vi "RP Lockin Batch Sweeper.vi"(6 "Samples per read":i32=1024, 8 "Error In":errorcluster, 9 "Dwell time":dbl=0.01, 10 "Frequencies":dbl[](array[numeric]), 11 "connection ID":refnum<k5>) -> (0 "Error Out":errorcluster, 1 "Y":dbl[](array[numeric]), 2 "X":dbl[](array[numeric]), 3 "connection ID out":refnum<k5>, 4 "F":dbl[](array[numeric]))   [LabVIEW 2015]
panel:
  out "32bit integer":i32
  out "Fifo cnt":i32
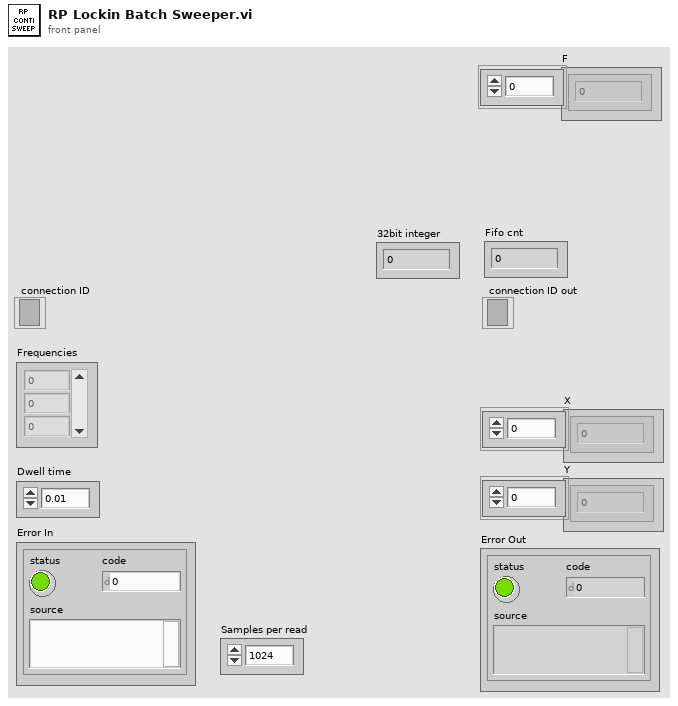
[diagram p1: front panel]
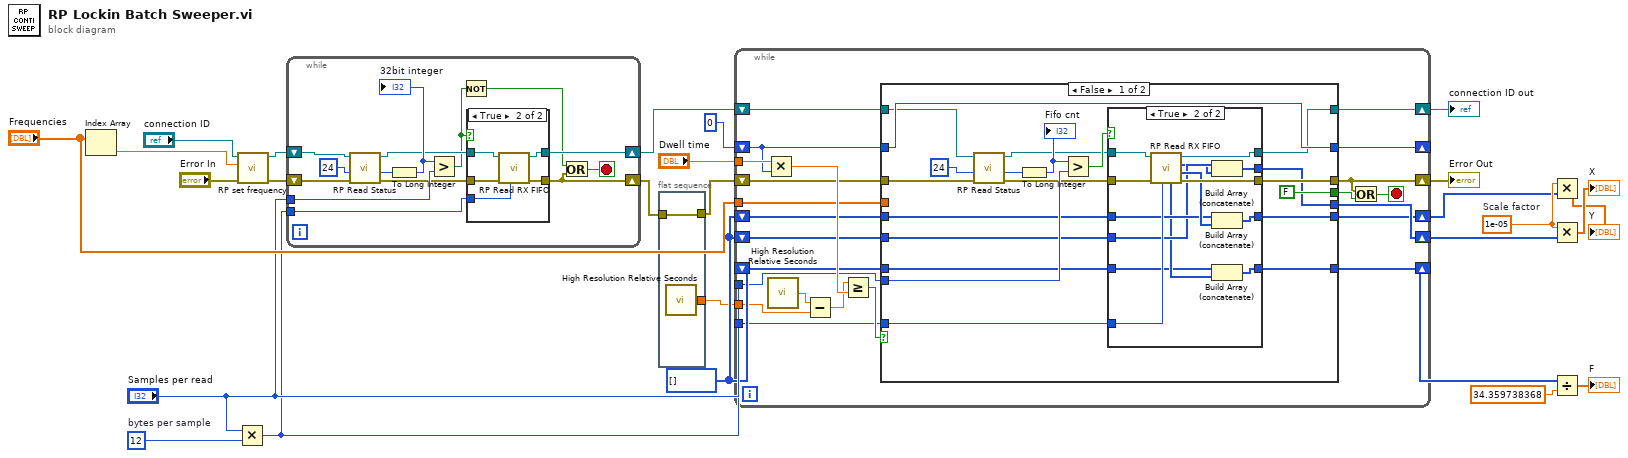
[diagram p0: block diagram]
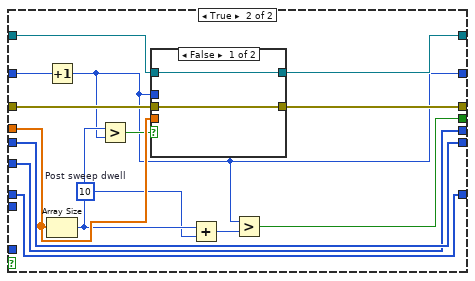
[diagram p4: hidden frame]
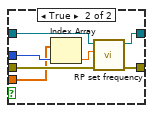
[diagram p5: hidden frame]
diagram:
  w12 = 1e-05  # Scale factor
  w9 = i32[] [] ("x*y")
  w20 = 12  # bytes per sample
  n1 = Index Array(array="Frequencies") -> (element=w24:dbl)  [unwired: 1 in]
  n2 = Multiply(x="Samples per read", y=w20) -> (x*y=w13:i32)
  n3 = call "RP set frequency.vi"("Error In"="Error In", "Frequency"=w24, "connection ID"="connection ID") -> ("Error Out"=w14:errorcluster, "connection ID out"=w16:refnum<k5>)  [unwired: 6 in, 1 out]
  n4 = while {
    tunnel: "Samples per read" -> [w37]
    shift-right: [w27] -> w3
    shift-left: w14 -> [w34]
    shift-right: [w32] -> w15
    shift-left: w16 -> [w33]
    tunnel: w13 -> [w31]
    stop <- w30 stop-if-true
    n5 = call "RP Read Status.vi"("Error In"=w34, "Status offset"=u64 24, "connection ID"=w33) -> ("Error Out"=w29:errorcluster, "Status response"=w38:u32, "connection ID out"=w36:refnum<k5>)  [unwired: 6 in]
    n6 = To Long Integer(number=w38) -> (32bit integer=w39:i32)
    "32bit integer" <- w39
    n7 = Greater?(x=w39, y=w37) -> (0:w35:bool)
    n8 = Not(x=w35) -> (.not. x?=w28:bool)
    n9 = case shown="True" w35 {
      tunnel: w36 -> [w42 w47]
      tunnel: w29 -> [w41 w46]
      tunnel: [w41 w45] -> w27
      tunnel: [w42 w44] -> w32
      tunnel: w31 -> [_ w43]
      frame False {
      }
      frame True {
        n10 = call "RP Read RX FIFO.vi"("FIFO Bytes per read"=w43, "Error In"=w46, "connection ID"=w47) -> ("Error Out"=w45:errorcluster, "connection ID out"=w44:refnum<k5>)  [unwired: 4 in, 3 out]
      }
    }
    n11 = Or(x=w28, y=w27) -> (x .or. y?=w30:bool)
  }
  n12 = flat-sequence {
    tunnel: w3 -> [w49]
    tunnel: [w49] -> w2
    tunnel: [w48] -> w1
    frame #0 {
      n13 = call <vilib>:"High Resolution Relative Seconds.vi"() -> ("relative seconds"=w48:dbl)
    }
  }
  n14 = while {
    shift-right: [w64] -> _
    shift-left: 0 -> [w66]
    tunnel: "Dwell time" -> [w72]
    tunnel: w1 -> [w68]
    tunnel: "Frequencies" -> [w65]
    shift-right: [w61] -> w10
    shift-left: w9 -> [w53]
    shift-right: [w52] -> w11
    shift-left: w9 -> [w60]
    tunnel: "Samples per read" -> [w63]
    tunnel: w13 -> [w62]
    shift-right: [w54] -> w18
    shift-left: w2 -> [w59]
    shift-right: [w57] -> w19
    shift-left: w15 -> [w58]
    shift-right: [w50] -> w7
    shift-left: w9 -> [w51]
    stop <- w55 stop-if-true
    n15 = Multiply(x=w72, y=w66) -> (x*y=w71:dbl)
    n16 = call <vilib>:"High Resolution Relative Seconds.vi"() -> ("relative seconds"=w70:dbl)
    n17 = Subtract(x=w70, y=w68) -> (x-y=w69:dbl)
    n18 = Greater Or Equal?(x=w69, y=w71) -> (x >= y?=w67:bool)
    n19 = case shown="False" w67 {
      tunnel: w66 -> [w92 w126]
      tunnel: w65 -> [_ w121]
      tunnel: [w92 w115] -> w64
      tunnel: w63 -> [w89 _]
      tunnel: w62 -> [w88 _]
      tunnel: [w75 w112] -> w61
      tunnel: w60 -> [w84 w119]
      tunnel: [w83 w119] -> w52
      tunnel: w59 -> [w82 w125]
      tunnel: [w80 w124] -> w54
      tunnel: w58 -> [w79 w123]
      tunnel: [w78 w122] -> w57
      tunnel: [FALSE w113] -> w56
      tunnel: w53 -> [w76 w112]
      tunnel: w51 -> [w74 w118]
      tunnel: [w73 w118] -> w50
      frame False {
        n20 = call "RP Read Status.vi"("Error In"=w82, "Status offset"=u64 24, "connection ID"=w79) -> ("Error Out"=w81:errorcluster, "Status response"=w90:u32, "connection ID out"=w85:refnum<k5>)  [unwired: 6 in]
        n21 = To Long Integer(number=w90) -> (32bit integer=w87:i32)
        "Fifo cnt" <- w87
        n22 = Greater?(x=w87, y=w89) -> (0:w86:bool)
        n23 = case shown="True" w86 {
          tunnel: w88 -> [_ w111]
          tunnel: w85 -> [w95 w110]
          tunnel: [w93 w101] -> w75
          tunnel: w84 -> [w97 w104]
          tunnel: [w97 w105] -> w83
          tunnel: w81 -> [w96 w109]
          tunnel: [w96 w108] -> w80
          tunnel: [w95 w107] -> w78
          tunnel: w76 -> [w93 w103]
          tunnel: w74 -> [w94 w99]
          tunnel: [w94 w98] -> w73
          frame False {
          }
          frame True {
            n24 = call "RP Read RX FIFO.vi"("FIFO Bytes per read"=w111, "Error In"=w109, "connection ID"=w110) -> ("Error Out"=w108:errorcluster, "Y"=w106:i32[], "X"=w102:i32[], "connection ID out"=w107:refnum<k5>, "F"=w100:i32[])  [unwired: 4 in]
            n25 = Build Array (concatenate)(w103, w102) -> (w101:i32[])
            n26 = Build Array (concatenate)(w104, w106) -> (w105:i32[])
            n27 = Build Array (concatenate)(w99, w100) -> (w98:i32[])
          }
        }
      }
      frame True {
        w116 = 10  # Post sweep dwell
        n28 = Increment(x=w126) -> (x+1=w115:i32)
        n29 = Array Size(array=w121) -> (size(s)=w117:i32)
        n30 = Greater?(x=w117, y=w115) -> (0:w120:bool)
        n31 = case shown="False" w120 {
          tunnel: w115 -> [_ w134]
          tunnel: w125 -> [w127 w133]
          tunnel: [w127 w132] -> w124
          tunnel: w123 -> [w128 w131]
          tunnel: [w128 w130] -> w122
          tunnel: w121 -> [_ w129]
          frame False {
          }
          frame True {
            n32 = Index Array(array=w129, index=w134) -> (element=w135:dbl)
            n33 = call "RP set frequency.vi"("Error In"=w133, "Frequency"=w135, "connection ID"=w131) -> ("Error Out"=w132:errorcluster, "connection ID out"=w130:refnum<k5>)  [unwired: 6 in, 1 out]
          }
        }
        n34 = Add(x=w117, y=w116) -> (x+y=w114:i32)
        n35 = Greater?(x=w115, y=w114) -> (0:w113:bool)
      }
    }
    n36 = Or(x=w54, y=w56) -> (x .or. y?=w55:bool)
  }
  "connection ID out" <- w19
  "Error Out" <- w18
  n37 = Multiply(x=w12, y=w11) -> (x*y=→"Y":dbl[])
  n38 = Multiply(x=w12, y=w10) -> (x*y=→"X":dbl[])
  n39 = Divide(x=w7, y=34.359738368 ("x*y")) -> (x/y=→"F":dbl[])
